vi "Final Count.vi"(8 "error in (no error)":errorcluster, 10 "event data":bool[](array[boolean]), 11 "GUI DigitalCount in":refnum<class "GUI DigitalCount.lvclass">) -> (0 "error out":errorcluster, 3 "GUI DigitalCount out":refnum<class "GUI DigitalCount.lvclass">)   [LabVIEW 2020, in "GUI DigitalCount.lvlib" / "GUI DigitalCount.lvclass"]
uses:
  GUI DigitalCount.lvclass
  GUI DigitalCount.lvclass/GUI DigitalCount.ctl
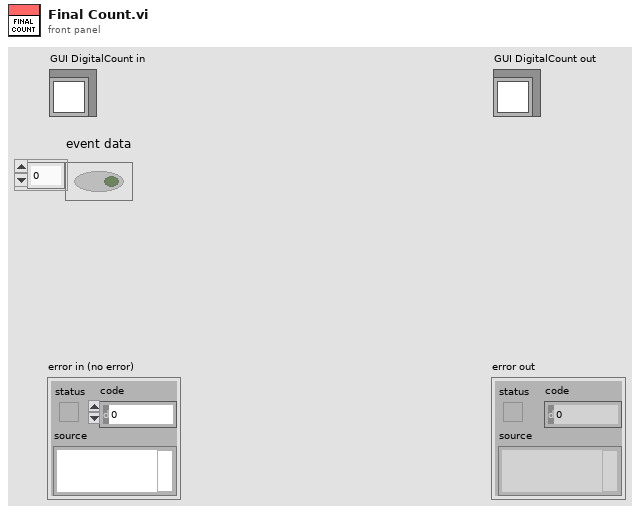
[diagram p1: front panel]
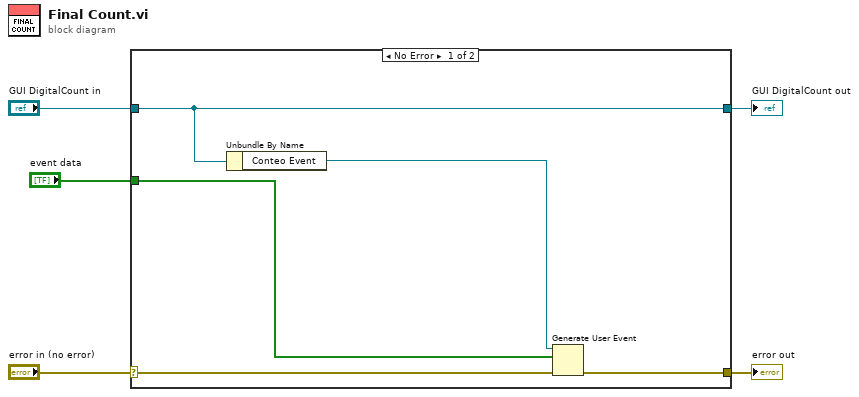
[diagram p0: block diagram]
diagram:
  n1 = case shown="No Error" "error in (no error)" {
    selector: "error in (no error)" -> [w10 w12]
    tunnel: [w8 w12] -> w4
    tunnel: [w9 w11] -> w2
    tunnel: "GUI DigitalCount in" -> [w9 w11]
    tunnel: "event data" -> [w6 _]
    frame No Error {
      n2 = Unbundle By Name(w9) -> ("Conteo Event"=w7:refnum<user-event>)
      n3 = Generate User Event(user event=w7, event data cluster=w6, error in=w10) -> (error out=w8:errorcluster)  [unwired: 1 in, 1 out]
    }
    frame Error {
    }
  }
  "error out" <- w4
  "GUI DigitalCount out" <- w2
